vi "Update XControl Based on Arrow Key Input.vi"(6 "PlatMods":T5, 9 "VKey":T6, 10 "Refnums for Resizing and Alignment in":T1, 11 "display state in":T2={"Graph Visible Items"={"Plot Legend"=FALSE, "Scale Legend"=FALSE, "Graph Palette"=FALSE, "Cursor Legend"=FALSE, "X Scrollbar"=FALSE}, "View Table"=FALSE, "Table Visible Items"={"Vertical Scrollbar"=FALSE, "Horizontal Scrollbar"=FALSE, "Row Headers"=FALSE, "Column Headers"=FALSE, "Vertical Lines"=FALSE, "Horizontal Lines"=FALSE}, "Header Font"={"Font Name"="", "Size"=0, "Bold"=FALSE, "Italic"=FALSE, "Underline"=FALSE, "Strikeout"=FALSE, "Color"=0}, "Cell Font"={"Font Name"="", "Size"=0, "Bold"=FALSE, "Italic"=FALSE, "Underline"=FALSE, "Strikeout"=FALSE, "Color"=0}, "Description and Tip..."={"Description"="", "Tip"=""}, "Moveable Splitter Position"=0, "Measurement Cursor Configuration"={"relative to t0"={"enable relative time"=FALSE, "Relative times (DT)"=[], "color"=0}, "range"={"enable range"=FALSE, "T1"=0.0, "T2"=0.0, "Fixed interval (T2-T1)"=0.0, "T1 color"=0, "T2 color"=0, "enable shading"=FALSE}, "periodic"={"enable periodic"=FALSE, "First event (E1)"=0.0, "Number events (Ei)"=0, "Event spacing (s)"=0.0, "First color"=0, "Events color"=0}, "absolute timestamp"={"enable absolute"=FALSE, "Timestamps (TS)"=[], "color"=0}}, "X Increment"=0.0, "X Scale"={"Label Visible"=FALSE, "Label Text"="", "Time Mode"=enum."Relative", "Format String"=""}, "Y Scale"={"Label Visible"=FALSE, "Label Text"="", "Scaling"=enum."Engineering Units", "Format String"=""}, "Colors"={"background"=16777215, "major grid"=8355711, "minor grid"=12632256, "font"=0}, "Cursors"={"List"=[], "Tags"=[]}, "Plots"=[], "Plot Color Wheel"=[3381759, 32768, 982784, 4375295, 13827953, 13457919, 16757522, 4343295, 16728758, 12095254], "registered user events"=variant} caption="State") -> (0 "Position.X":dbl, 1 "selected cursor":string, 2 "Refnums for Resizing and Alignment out":T1, 3 "display state out":T2={"Graph Visible Items"={"Plot Legend"=FALSE, "Scale Legend"=FALSE, "Graph Palette"=FALSE, "Cursor Legend"=FALSE, "X Scrollbar"=FALSE}, "View Table"=FALSE, "Table Visible Items"={"Vertical Scrollbar"=FALSE, "Horizontal Scrollbar"=FALSE, "Row Headers"=FALSE, "Column Headers"=FALSE, "Vertical Lines"=FALSE, "Horizontal Lines"=FALSE}, "Header Font"={"Font Name"="", "Size"=0, "Bold"=FALSE, "Italic"=FALSE, "Underline"=FALSE, "Strikeout"=FALSE, "Color"=0}, "Cell Font"={"Font Name"="", "Size"=0, "Bold"=FALSE, "Italic"=FALSE, "Underline"=FALSE, "Strikeout"=FALSE, "Color"=0}, "Description and Tip..."={"Description"="", "Tip"=""}, "Moveable Splitter Position"=0, "Measurement Cursor Configuration"={"relative to t0"={"enable relative time"=FALSE, "Relative times (DT)"=[], "color"=0}, "range"={"enable range"=FALSE, "T1"=0.0, "T2"=0.0, "Fixed interval (T2-T1)"=0.0, "T1 color"=0, "T2 color"=0, "enable shading"=FALSE}, "periodic"={"enable periodic"=FALSE, "First event (E1)"=0.0, "Number events (Ei)"=0, "Event spacing (s)"=0.0, "First color"=0, "Events color"=0}, "absolute timestamp"={"enable absolute"=FALSE, "Timestamps (TS)"=[], "color"=0}}, "X Increment"=0.0, "X Scale"={"Label Visible"=FALSE, "Label Text"="", "Time Mode"=enum."Relative", "Format String"=""}, "Y Scale"={"Label Visible"=FALSE, "Label Text"="", "Scaling"=enum."Engineering Units", "Format String"=""}, "Colors"={"background"=16777215, "major grid"=8355711, "minor grid"=12632256, "font"=0}, "Cursors"={"List"=[], "Tags"=[]}, "Plots"=[], "Plot Color Wheel"=[3381759, 32768, 982784, 4375295, 13827953, 13457919, 16757522, 4343295, 16728758, 12095254], "registered user events"=variant} caption="State", 4 "discard?":bool)   [LabVIEW 2017, in "Waveforms with Cursors.xctl"]
doc: "On left/right arrow, move the selected cursor and update the table value.\nOn up/down arrow, increment the cursor selection."
uses:
  <vilib>/addons/_XControls/Waveforms with Cursors/Waveforms with Cursors.xctl
  <vilib>/addons/_XControls/Waveforms with Cursors/Controls/Refnums Typedef.ctl
  <vilib>/event_ctls.llb/eventvkey.ctl
  <vilib>/addons/_XControls/Waveforms with Cursors/Controls/State.ctl
  <vilib>/Utility/miscctls.llb/LVFontTypeDef.ctl
  <vilib>/addons/_XControls/Waveforms with Cursors/Controls/Waveform Cursor Configuration.ctl
  <vilib>/Utility/miscctls.llb/LVRowAndColumnTypeDef.ctl
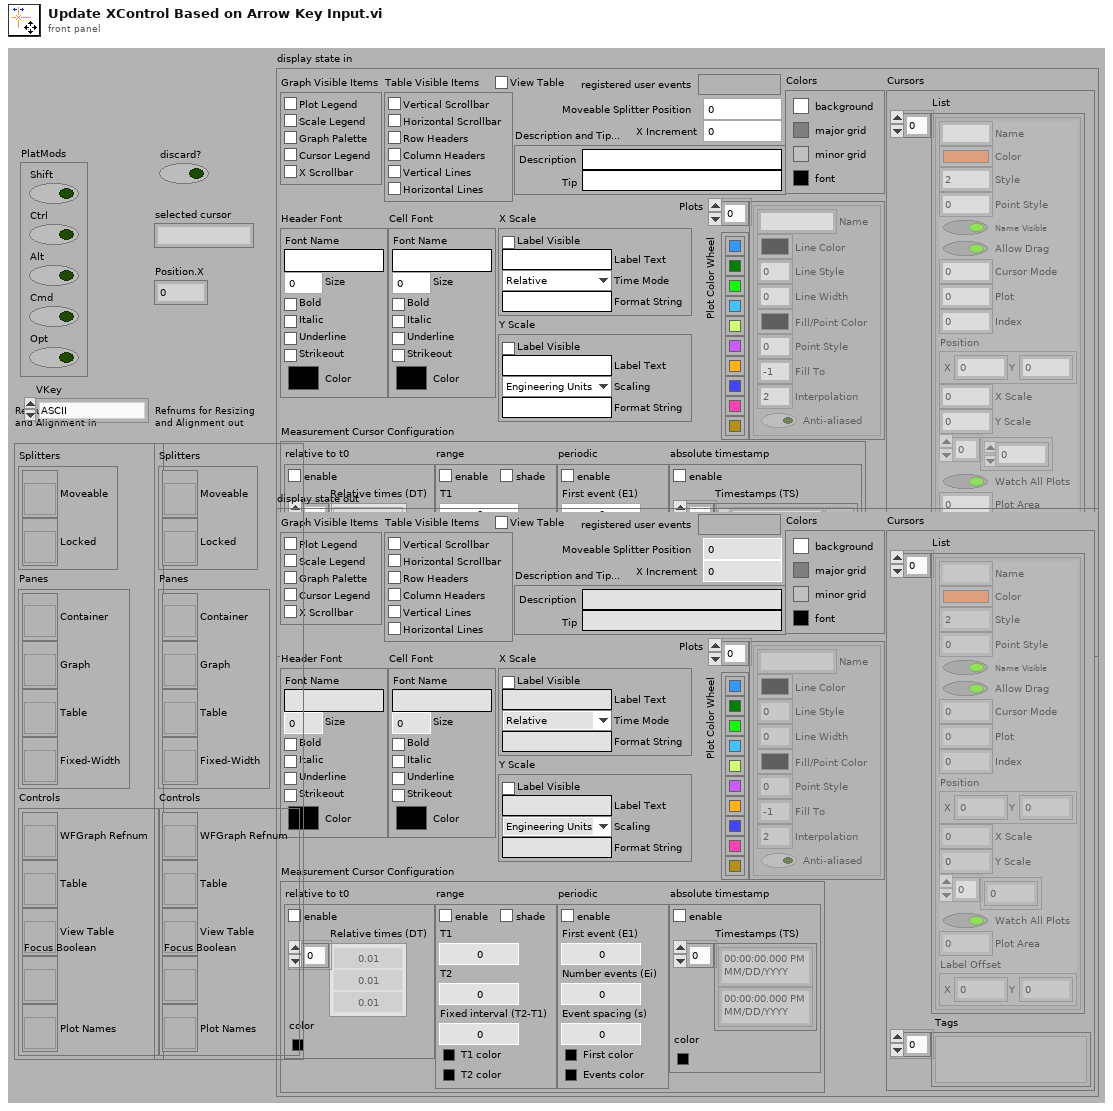
[diagram p1: front panel]
types:
  T1 = typedef "Waveforms with Cursors.xctl/Refnums Typedef.ctl" = cluster{"Splitters":cluster{"Moveable":refnum<vi>, "Locked":refnum<vi>}, "Panes":cluster{"Container":refnum<vi>, "Graph":refnum<vi>, "Table":refnum<vi>, "Fixed-Width":refnum<vi>}, "Controls":cluster{"WFGraph Refnum":refnum<vi>, "Table":refnum<vi>, "View Table":refnum<vi>, "Focus Boolean":refnum<vi>, "Plot Names":refnum<vi>}}
  T2 = typedef "Waveforms with Cursors.xctl/State.ctl" = cluster{"Graph Visible Items":cluster{"Plot Legend":bool, "Scale Legend":bool, "Graph Palette":bool, "Cursor Legend":bool, "X Scrollbar":bool}, "View Table":bool, "Table Visible Items":cluster{"Vertical Scrollbar":bool, "Horizontal Scrollbar":bool, "Row Headers":bool, "Column Headers":bool, "Vertical Lines":bool, "Horizontal Lines":bool}, "Header Font":T3, "Cell Font":T3, "Description and Tip...":cluster{"Description":string, "Tip":string}, "Moveable Splitter Position":i32, "Measurement Cursor Configuration":T4, "X Increment":dbl, "X Scale":cluster{"Label Visible":bool, "Label Text":string, "Time Mode":enum16{"Relative", "Absolute"}, "Format String":string}, "Y Scale":cluster{"Label Visible":bool, "Label Text":string, "Scaling":enum16{"Engineering Units", "Voltage"}, "Format String":string}, "Colors":cluster{"background":u32, "major grid":u32, "minor grid":u32, "font":u32}, "Cursors":cluster{"List":cluster{"Name":string, "Color":u32, "Style":i32, "Point Style":u8, "Name Visible":bool, "Allow Drag":bool, "Cursor Mode":u32, "Plot":i32, "Index":i32, "Position":cluster{"X":dbl, "Y":dbl}, "X Scale":u32, "Y Scale":u32, "Watch Plots":i32[], "Watch All Plots":bool, "Plot Area":i32, "Label Offset":cluster{"X":dbl, "Y":dbl}}[], "Tags":variant[]}, "Plots":cluster{"Name":string, "Line Color":u32, "Line Style":u8, "Line Width":u8, "Fill/Point Color":u32, "Point Style":u8, "Fill To":i16, "Interpolation":u8, "Anti-aliased":bool}[], "Plot Color Wheel":u32[], "registered user events":variant}
  T3 = typedef "LVFontTypeDef.ctl" = cluster{"Font Name":string, "Size":u16, "Bold":bool, "Italic":bool, "Underline":bool, "Strikeout":bool, "Color":u32}
  T4 = typedef "Waveforms with Cursors.xctl/Waveform Cursor Configuration.ctl" = cluster{"relative to t0":cluster{"enable relative time":bool, "Relative times (DT)":dbl[], "color":u32}, "range":cluster{"enable range":bool, "T1":dbl, "T2":dbl, "Fixed interval (T2-T1)":dbl, "T1 color":u32, "T2 color":u32, "enable shading":bool}, "periodic":cluster{"enable periodic":bool, "First event (E1)":dbl, "Number events (Ei)":i32, "Event spacing (s)":dbl, "First color":u32, "Events color":u32}, "absolute timestamp":cluster{"enable absolute":bool, "Timestamps (TS)":timestamp[], "color":u32}}
  T5 = cluster{"Shift":bool, "Ctrl":bool, "Alt":bool, "Cmd":bool, "Opt":bool}
  T6 = typedef "eventvkey.ctl" = enum16{"ASCII", "Enter", "Return", "Shift", "Ctrl", "Alt", "Cmd", "Opt", "Caps", "NumLock", "Clear", "Break", "Up", "Down", "Left", "Right", "Insert", "Delete", "Home", "End", "PageUp", "PageDown", "Escape", "Help", "Pause", "ScrollLock", "F1", "F2", "F3", "F4", "F5", "F6", "F7", "F8", "F9", "F10", "F11", "F12", "F13", "F14", "F15", "F16", "F17", "F18", "F19", "F20", "F21", "F22", "F23", "F24", "Play", "VolumeUp", "VolumeDown", "Mute", "Two Byte Char"}
  T7 = typedef "LVRowAndColumnTypeDef.ctl" = cluster{"Row":i32, "Column":i32}
  T8 = cluster{"Name":string, "Color":u32, "Style":i32, "Point Style":u8, "Name Visible":bool, "Allow Drag":bool, "Cursor Mode":u32, "Plot":i32, "Index":i32, "Position":cluster{"X":dbl, "Y":dbl}, "X Scale":u32, "Y Scale":u32, "Watch Plots":i32[], "Watch All Plots":bool, "Plot Area":i32, "Label Offset":cluster{"X":dbl, "Y":dbl}}[]
  T9 = cluster{"Name":string, "Color":u32, "Style":i32, "Point Style":u8, "Name Visible":bool, "Allow Drag":bool, "Cursor Mode":u32, "Plot":i32, "Index":i32, "Position":cluster{"X":dbl, "Y":dbl}, "X Scale":u32, "Y Scale":u32, "Watch Plots":i32[], "Watch All Plots":bool, "Plot Area":i32, "Label Offset":cluster{"X":dbl, "Y":dbl}}
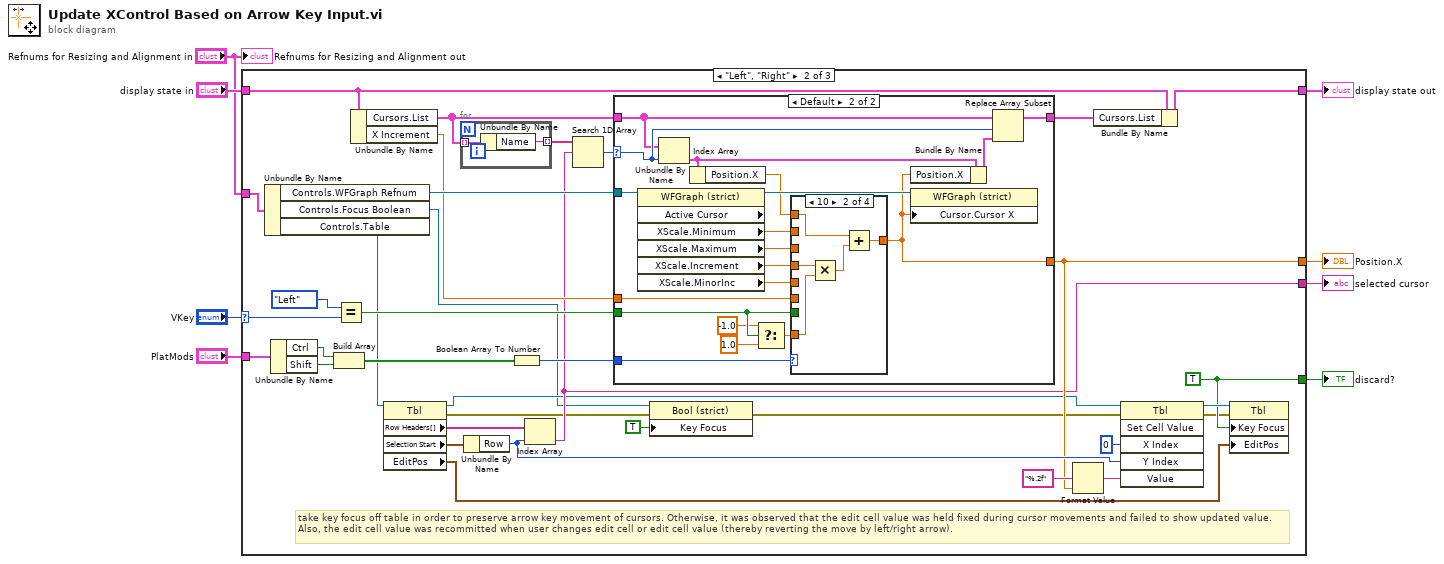
[diagram p0: block diagram]
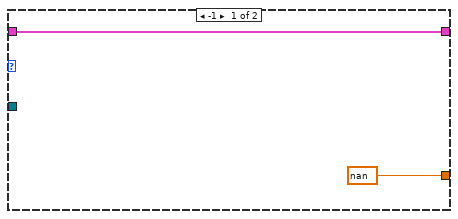
[diagram p3: hidden frame]
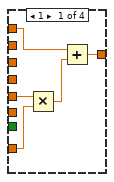
[diagram p4: hidden frame]
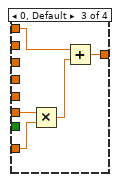
[diagram p5: hidden frame]
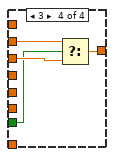
[diagram p6: hidden frame]
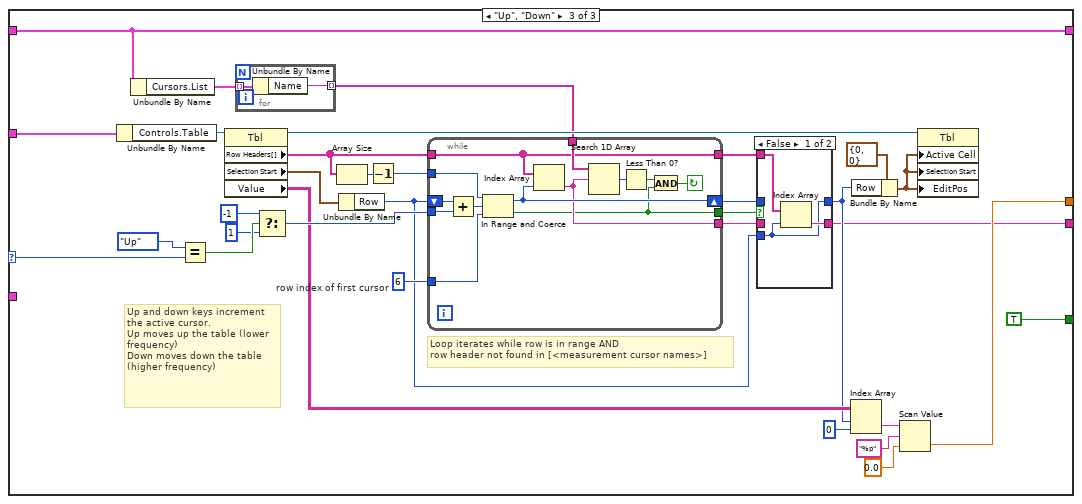
[diagram p7: hidden frame]
diagram:
  n1 = case shown="\"Left\", \"Right\"" "VKey" {
    selector: "VKey" -> [_ w42 w118]
    tunnel: [_ w22 TRUE] -> w8
    tunnel: "PlatMods" -> [_ w39 _]
    tunnel: "Refnums for Resizing and Alignment in" -> [_ w21 w88]
    tunnel: [_ w25 w106] -> w5
    tunnel: [_ w16 w91] -> w4
    tunnel: [w9 w17 w97] -> w3
    tunnel: "display state in" -> [w9 w18 w97]
    frame Default {
    }
    frame "Left", "Right" {
      w22 = TRUE
      # "take key focus off table in order to preserve arrow key movement of cursors. Otherwise, it was observed that the edit cell value was held fixed during cursor movements and failed to show updated value. Also, the edit cell value was recommitted when user changes edit cell or edit cell value (thereby reverting the move by left/right arrow)."
      n2 = Unbundle By Name(w21) -> ("Controls.WFGraph Refnum"=w36:refnum<vi>, "Controls.Focus Boolean"=w14:refnum<vi>, "Controls.Table"=w35:refnum<vi>)
      n3 = Unbundle By Name(w39) -> ("Ctrl"=w38:bool, "Shift"=w37:bool)
      n4 = Build Array(w38, w37) -> (w44:bool[])
      n5 = Equal?(x=eventvkey."Left" ("VKey"), y=w42) -> (x = y?=w41:bool)
      n6 = Unbundle By Name(w18) -> ("Cursors.List"=w20:T8, "X Increment"=w27:dbl)
      n7 = property class="Tbl"(reference=w35) -> (reference out=w15:refnum<vi>, error out=w13:errorcluster, "Row Headers[]"=w23:string[], "Selection Start"=w34:T7, "EditPos"=w28:T7)  [unwired: 1 in]
      n8 = for {
        tunnel: w20 -> [w86] mode=indexing
        tunnel: [w85] -> w26 mode=indexing
        n9 = Unbundle By Name(w86) -> ("Name"=w85:string)
      }
      n10 = Unbundle By Name(w34) -> ("Row"=w30:i32)
      n11 = Boolean Array To Number(Boolean array=w44) -> (number=w43:u32)
      n12 = Index Array(array=w23, index=w30) -> (element=w16:string)
      n13 = Search 1D Array(1D array=w26, element=w16) -> (index of element=w24:i32)  [unwired: 1 in]
      n14 = case shown="Default" w24 {
        selector: w24 -> [_ w51]
        tunnel: w43 -> [_ w64]
        tunnel: w41 -> [_ w59]
        tunnel: w36 -> [_ w55]
        tunnel: w27 -> [_ w53]
        tunnel: [nan ("XScale.Maximum") w52] -> w25
        tunnel: w20 -> [w45 w48]
        tunnel: [w45 w47] -> w19
        frame -1 {
        }
        frame Default {
          n15 = property class="WFGraph (strict)" props=["Active Cursor", "XScale", "Minimum", "XScale", "Maximum", "XScale", "Increment", "XScale", "MinorInc"](reference=w55) -> (reference out=w65:refnum<vi>, "XScale.Minimum"=w63:dbl, "XScale.Maximum"=w62:dbl, "XScale.Increment"=w61:dbl, "XScale.MinorInc"=w60:dbl)  [unwired: 1 in, 2 out]
          n16 = Index Array(array=w48, index=w51) -> (element=w50:T9)
          n17 = Unbundle By Name(w50) -> ("Position.X"=w49:dbl)
          n18 = Select(t=-1.0, s=w59, f=1.0) -> (s? t:f=w56:dbl)
          n19 = case shown="10" w64 {
            tunnel: w59 -> [_ _ _ w82]
            tunnel: w63 -> [_ _ _ w84]
            tunnel: w62 -> [_ _ _ w83]
            tunnel: [w68 w71 w77 w81] -> w52
            tunnel: w61 -> [_ w74 _ _]
            tunnel: w60 -> [w70 _ _ _]
            tunnel: w49 -> [w67 w72 w78 _]
            tunnel: w56 -> [w69 w73 w79 _]
            tunnel: w53 -> [_ _ w76 _]
            frame 1 {
              n20 = Multiply(x=w70, y=w69) -> (x*y=w66:dbl)
              n21 = Add(x=w67, y=w66) -> (x+y=w68:dbl)
            }
            frame 2 {
              n22 = Multiply(x=w74, y=w73) -> (x*y=w75:dbl)
              n23 = Add(x=w72, y=w75) -> (x+y=w71:dbl)
            }
            frame 0, Default {
              n24 = Multiply(x=w76, y=w79) -> (x*y=w80:dbl)
              n25 = Add(x=w78, y=w80) -> (x+y=w77:dbl)
            }
            frame 3 {
              n26 = Select(t=w84, s=w82, f=w83) -> (s? t:f=w81:dbl)
            }
          }
          n27 = Bundle By Name(cluster=w50, "Position.X"=w52) -> (w54:T9)
          n28 = property class="WFGraph (strict)"(reference=w65, "Cursor.Cursor X"=w52) -> ()  [unwired: 1 in, 2 out]
          n29 = Replace Array Subset(array=w48, new element=w54, index=w51) -> (w47:T8)
        }
      }
      n30 = property class="Bool (strict)"(reference=w14, error in=w13, "Key Focus"=TRUE) -> (error out=w12:errorcluster)  [unwired: 1 out]
      n31 = Format Value(format string="%.2f", value (0)=w25) -> (output string=w32:string)  [unwired: 1 in]
      n32 = Bundle By Name(cluster=w18, "Cursors.List"=w19) -> (w17:T2)
      n33 = invoke class="Tbl" method="Set Cell Value"(reference=w15, error in=w12, "X Index"=u32 0, "Y Index"=w30, "Value"=w32) -> (reference out=w29:refnum<vi>, error out=w11:errorcluster)  [unwired: 1 in, 4 out]
      n34 = property class="Tbl"(reference=w29, error in=w11, "Key Focus"=w22, "EditPos"=w28) -> ()  [unwired: 2 out]
    }
    frame "Up", "Down" {
      w98 = 6  # row index of first cursor
      # "Loop iterates while row is in range AND \nrow header not found in [<measurement cursor names>]"
      # "Up and down keys increment the active cursor.\nUp moves up the table (lower frequency)\nDown moves down the table (higher frequency)"
      n35 = Unbundle By Name(w88) -> ("Controls.Table"=w113:refnum<vi>)
      n36 = Unbundle By Name(w97) -> ("Cursors.List"=w96:T8)
      n37 = Equal?(x=eventvkey."Up" ("VKey"), y=w118) -> (x = y?=w116:bool)
      n38 = property class="Tbl"(reference=w113) -> (reference out=w117:refnum<vi>, "Row Headers[]"=w99:string[], "Selection Start"=w100:T7, "Value"=w105:string[][])  [unwired: 1 in, 1 out]
      n39 = for {
        tunnel: w96 -> [w139] mode=indexing
        tunnel: [w138] -> w95 mode=indexing
        n40 = Unbundle By Name(w139) -> ("Name"=w138:string)
      }
      n41 = Select(t=-1 ("lower limit"), s=w116, f=1 ("lower limit")) -> (s? t:f=w110:i32)
      n42 = Array Size(array=w99) -> (size(s)=w115:i32)
      n43 = Unbundle By Name(w100) -> ("Row"=w87:i32)
      n44 = Decrement(x=w115) -> (x-1=w103:i32)
      n45 = while {
        tunnel: w103 -> [w137]
        tunnel: w110 -> [w136]
        tunnel: w99 -> [w125]
        tunnel: [w130] -> w90
        shift-right: [w133] -> w92
        shift-left: w87 -> [w134]
        tunnel: w98 -> [w127]
        tunnel: w95 -> [w132]
        tunnel: [w126] -> w94
        tunnel: [w125] -> w89
        stop <- w131 continue-if-true
        n46 = Add(x=w134, y=w136) -> (x+y=w135:i32)
        n47 = In Range and Coerce(upper limit=w137, x=w135, lower limit=w127) -> (coerced(x)=w133:i32, In Range?=w126:bool)
        n48 = Index Array(array=w125, index=w133) -> (element=w130:string)
        n49 = Search 1D Array(1D array=w132, element=w130) -> (index of element=w129:i32)  [unwired: 1 in]
        n50 = Less Than 0?(x=w129) -> (x < 0?=w128:bool)
        n51 = And(x=w128, y=w126) -> (x .and. y?=w131:bool)
      }
      n52 = case shown="False" w94 {
        tunnel: [w120 w124] -> w93
        tunnel: w92 -> [_ w124]
        tunnel: [w121 w123] -> w91
        tunnel: w90 -> [_ w123]
        tunnel: w87 -> [w120 _]
        tunnel: w89 -> [w122 _]
        frame False {
          n53 = Index Array(array=w122, index=w120) -> (element=w121:string)
        }
        frame True {
        }
      }
      n54 = Index Array(array=w105, index (row)=w93, index (col)=0 ("disabled index (col)")) -> (element=w109:string)
      n55 = Bundle By Name(cluster=T7 {"Row"=0, "Column"=0} ("Active Cell:Active Cell"), "Row"=w93) -> (w101:T7)
      n56 = Scan Value(string=w109, format string="%p", default (0 dbl)=0.0) -> (value=w106:dbl)  [unwired: 1 out]
      n57 = property class="Tbl"(reference=w117, "Active Cell"=w101, "Selection Start"=w101, "EditPos"=w101) -> ()  [unwired: 1 in, 2 out]
    }
  }
  "discard?" <- w8
  "Position.X" <- w5
  "selected cursor" <- w4
  "display state out" <- w3
  "Refnums for Resizing and Alignment out" <- "Refnums for Resizing and Alignment in"
